vi "Actor Core.vi"(8 "error in":errorcluster, 11 "DAQVoltage in":refnum<class "DAQVoltage.lvclass">) -> (0 "error out":errorcluster, 3 "Actor out":refnum<class "Actor.lvclass">)   [LabVIEW 2025, in "DAQVoltage.lvlib" / "DAQVoltage.lvclass"]
doc: "<p>(<strong>Filename</strong>: <span class=\"dnl\">Actor Framework.lvlib:Actor.lvclass:Actor Core.vi</span>)</p>\n<p>Receives messages to the actor, reacts to them, and initiates any error handling that may shut the actor down.</p>\n<p>Descendant classes may override this VI to append parallel tasks for the actor to complete while it handles messages. Overrides use the <a href=\"nihelplauncher://docs/csh?context=lvcore_glang_udclass\">Call Parent Class Method</a> node.</p>"
uses:
  DAQVoltage.lvclass
  DAQVoltage.lvclass/DAQVoltage.ctl
  <vilib>/ActorFramework/Actor/Actor.lvclass
  DAQVoltage Messages/register_voltage Msg/register_voltage Msg.lvclass
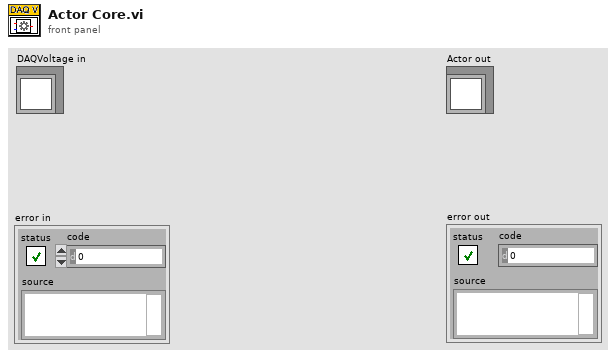
[diagram p1: front panel]
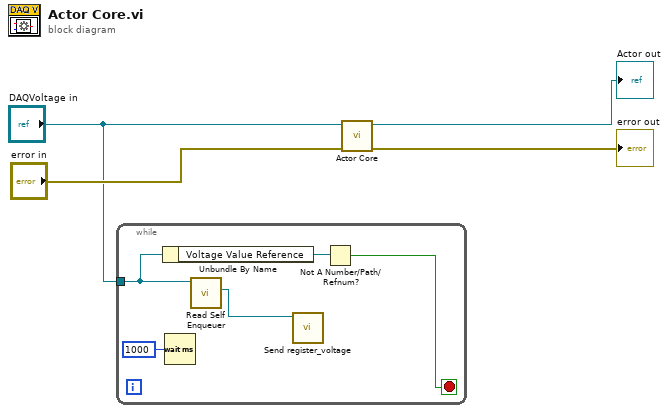
[diagram p0: block diagram]
diagram:
  n1 = while {
    tunnel: "DAQVoltage in" -> [w8]
    stop <- w6 stop-if-true
    n2 = Unbundle By Name(w8) -> ("Voltage Value Reference"=w7:refnum<data-value>)
    n3 = Wait (ms)(milliseconds to wait=u32 1000) -> ()  [unwired: 1 out]
    n4 = call <vilib>:"Read Self Enqueuer.vi"("Actor"=w8) -> ("Self Enqueuer"=w5:refnum<class "Message Enqueuer.lvclass">)  [unwired: 10 in]
    n5 = call "Send register_voltage.vi"("Message Enqueuer"=w5) -> ()  [unwired: 9 in, 2 out]
    n6 = Not A Number/Path/Refnum?(number/path/refnum=w7) -> (NaN/Path/Refnum?=w6:bool)
  }
  n7 = call-parent "Actor Core.vi"("error in"="error in", "Actor in"="DAQVoltage in") -> ("error out"=→"error out":errorcluster, "Actor out"=→"Actor out":refnum<class "Actor.lvclass">)  [unwired: 8 in]
